vi "MeasureGrowthNotLog.vi"(10 "DaysBack":i32=7, 11 "Data":cluster{"Cases":i32[], "Days":timestamp[]}={"Cases"=[0, 0, 0, 0, 2, 2, 2, 2, 2, 3, 3, 3, 6, 6, 6, 6, 6, 6, 6, 6, 7, 7, 8, 8, 8, 8, 8, 8, 8, 8, 10, 10, 10, 10, 10, 10, 11, 11, 12, 12, 21, 25, 35, 51, 59, 102, 116, 167, 179, 247, 250, 305, 372, 480, 588, 741, 892, 1065, 1289, 1524, 1826, 2253, 2641, 3176, 4035, 4863, 5671, 6352, 7412, 8570, 9939, 11170, 12563, 13886], "Days"=[timestamp(3662524800 s since 1904-01-01), timestamp(3662611200 s since 1904-01-01), timestamp(3662697600 s since 1904-01-01), timestamp(3662784000 s since 1904-01-01), timestamp(3662870400 s since 1904-01-01), timestamp(3662956800 s since 1904-01-01), timestamp(3663043200 s since 1904-01-01), timestamp(3663129600 s since 1904-01-01), timestamp(3663216000 s since 1904-01-01), timestamp(3663302400 s since 1904-01-01), timestamp(3663388800 s since 1904-01-01), timestamp(3663475200 s since 1904-01-01), timestamp(3663561600 s since 1904-01-01), timestamp(3663648000 s since 1904-01-01), timestamp(3663734400 s since 1904-01-01), timestamp(3663820800 s since 1904-01-01), timestamp(3663907200 s since 1904-01-01), timestamp(3663993600 s since 1904-01-01), timestamp(3664080000 s since 1904-01-01), timestamp(3664166400 s since 1904-01-01), timestamp(3664252800 s since 1904-01-01), timestamp(3664339200 s since 1904-01-01), timestamp(3664425600 s since 1904-01-01), timestamp(3664512000 s since 1904-01-01), timestamp(3664598400 s since 1904-01-01), timestamp(3664684800 s since 1904-01-01), timestamp(3664771200 s since 1904-01-01), timestamp(3664857600 s since 1904-01-01), timestamp(3664944000 s since 1904-01-01), timestamp(3665030400 s since 1904-01-01), timestamp(3665116800 s since 1904-01-01), timestamp(3665203200 s since 1904-01-01), timestamp(3665289600 s since 1904-01-01), timestamp(3665376000 s since 1904-01-01), timestamp(3665462400 s since 1904-01-01), timestamp(3665548800 s since 1904-01-01), timestamp(3665635200 s since 1904-01-01), timestamp(3665721600 s since 1904-01-01), timestamp(3665808000 s since 1904-01-01), timestamp(3665894400 s since 1904-01-01), timestamp(3665980800 s since 1904-01-01), timestamp(3666067200 s since 1904-01-01), timestamp(3666153600 s since 1904-01-01), timestamp(3666240000 s since 1904-01-01), timestamp(3666326400 s since 1904-01-01), timestamp(3666412800 s since 1904-01-01), timestamp(3666499200 s since 1904-01-01), timestamp(3666585600 s since 1904-01-01), timestamp(3666672000 s since 1904-01-01), timestamp(3666758400 s since 1904-01-01), timestamp(3666844800 s since 1904-01-01), timestamp(3666931200 s since 1904-01-01), timestamp(3667017600 s since 1904-01-01), timestamp(3667104000 s since 1904-01-01), timestamp(3667190400 s since 1904-01-01), timestamp(3667276800 s since 1904-01-01), timestamp(3667363200 s since 1904-01-01), timestamp(3667449600 s since 1904-01-01), timestamp(3667536000 s since 1904-01-01), timestamp(3667622400 s since 1904-01-01), timestamp(3667708800 s since 1904-01-01), timestamp(3667795200 s since 1904-01-01), timestamp(3667881600 s since 1904-01-01), timestamp(3667968000 s since 1904-01-01), timestamp(3668054400 s since 1904-01-01), timestamp(3668140800 s since 1904-01-01), timestamp(3668227200 s since 1904-01-01), timestamp(3668313600 s since 1904-01-01), timestamp(3668400000 s since 1904-01-01), timestamp(3668486400 s since 1904-01-01), timestamp(3668572800 s since 1904-01-01), timestamp(3668659200 s since 1904-01-01), timestamp(3668745600 s since 1904-01-01), timestamp(3668832000 s since 1904-01-01)]}) -> (0 "Plot":T2(graph)=[{"Days"=[timestamp(3662524800 s since 1904-01-01), timestamp(3662611200 s since 1904-01-01), timestamp(3662697600 s since 1904-01-01), timestamp(3662784000 s since 1904-01-01), timestamp(3662870400 s since 1904-01-01), timestamp(3662956800 s since 1904-01-01), timestamp(3663043200 s since 1904-01-01), timestamp(3663129600 s since 1904-01-01), timestamp(3663216000 s since 1904-01-01), timestamp(3663302400 s since 1904-01-01), timestamp(3663388800 s since 1904-01-01), timestamp(3663475200 s since 1904-01-01), timestamp(3663561600 s since 1904-01-01), timestamp(3663648000 s since 1904-01-01), timestamp(3663734400 s since 1904-01-01), timestamp(3663820800 s since 1904-01-01), timestamp(3663907200 s since 1904-01-01), timestamp(3663993600 s since 1904-01-01), timestamp(3664080000 s since 1904-01-01), timestamp(3664166400 s since 1904-01-01), timestamp(3664252800 s since 1904-01-01), timestamp(3664339200 s since 1904-01-01), timestamp(3664425600 s since 1904-01-01), timestamp(3664512000 s since 1904-01-01), timestamp(3664598400 s since 1904-01-01), timestamp(3664684800 s since 1904-01-01), timestamp(3664771200 s since 1904-01-01), timestamp(3664857600 s since 1904-01-01), timestamp(3664944000 s since 1904-01-01), timestamp(3665030400 s since 1904-01-01), timestamp(3665116800 s since 1904-01-01), timestamp(3665203200 s since 1904-01-01), timestamp(3665289600 s since 1904-01-01), timestamp(3665376000 s since 1904-01-01), timestamp(3665462400 s since 1904-01-01), timestamp(3665548800 s since 1904-01-01), timestamp(3665635200 s since 1904-01-01), timestamp(3665721600 s since 1904-01-01), timestamp(3665808000 s since 1904-01-01), timestamp(3665894400 s since 1904-01-01), timestamp(3665980800 s since 1904-01-01), timestamp(3666067200 s since 1904-01-01), timestamp(3666153600 s since 1904-01-01), timestamp(3666240000 s since 1904-01-01), timestamp(3666326400 s since 1904-01-01), timestamp(3666412800 s since 1904-01-01), timestamp(3666499200 s since 1904-01-01), timestamp(3666585600 s since 1904-01-01), timestamp(3666672000 s since 1904-01-01), timestamp(3666758400 s since 1904-01-01), timestamp(3666844800 s since 1904-01-01), timestamp(3666931200 s since 1904-01-01), timestamp(3667017600 s since 1904-01-01), timestamp(3667104000 s since 1904-01-01), timestamp(3667190400 s since 1904-01-01), timestamp(3667276800 s since 1904-01-01), timestamp(3667363200 s since 1904-01-01), timestamp(3667449600 s since 1904-01-01), timestamp(3667536000 s since 1904-01-01), timestamp(3667622400 s since 1904-01-01), timestamp(3667708800 s since 1904-01-01), timestamp(3667795200 s since 1904-01-01), timestamp(3667881600 s since 1904-01-01), timestamp(3667968000 s since 1904-01-01), timestamp(3668054400 s since 1904-01-01), timestamp(3668140800 s since 1904-01-01), timestamp(3668227200 s since 1904-01-01), timestamp(3668313600 s since 1904-01-01), timestamp(3668400000 s since 1904-01-01), timestamp(3668486400 s since 1904-01-01), timestamp(3668572800 s since 1904-01-01), timestamp(3668659200 s since 1904-01-01), timestamp(3668745600 s since 1904-01-01), timestamp(3668832000 s since 1904-01-01)], "ConfirmedCases"=[0.0, 0.0, 0.0, 0.0, 0.0, 0.0, 0.0, 0.0, 0.0, 0.0, 0.0, 0.0, 0.0, 0.0, 0.0, 0.0, 0.0, 0.0, 0.0, 0.0, 0.0, 0.0, 0.0, 0.0, 0.0, 0.0, 0.0, 0.0, 0.0, 0.0, 0.0, 0.0, 0.0, 0.0, 0.0, 0.0, 0.0, 0.0, 0.0, 0.0, 0.0, 0.0, 1.0, 1.0, 1.0, 1.0, 1.0, 2.0, 3.0, 4.0, 4.0, 4.0, 4.0, 6.0, 11.0, 14.0, 17.0, 19.0, 24.0, 29.0, 33.0, 40.0, 52.0, 67.0, 83.0, 100.0, 121.0, 132.0, 149.0, 182.0, 212.0, 243.0, 282.0, 321.0]}, {"Days"=[timestamp(3668313600 s since 1904-01-01), timestamp(3668400000 s since 1904-01-01), timestamp(3668486400 s since 1904-01-01), timestamp(3668572800 s since 1904-01-01), timestamp(3668659200 s since 1904-01-01), timestamp(3668745600 s since 1904-01-01), timestamp(3668832000 s since 1904-01-01)], "ConfirmedCases"=[132.01823524302534, 153.55263572024907, 178.59966006386384, 207.73227646213113, 241.6169138771523, 281.0287070731711, 326.8692283660796]}, {"Days"=[timestamp(3668313600 s since 1904-01-01), timestamp(3668400000 s since 1904-01-01), timestamp(3668486400 s since 1904-01-01), timestamp(3668572800 s since 1904-01-01), timestamp(3668659200 s since 1904-01-01), timestamp(3668745600 s since 1904-01-01), timestamp(3668832000 s since 1904-01-01)], "ConfirmedCases"=[140.59609548662908, 162.8828644131387, 188.9766356577397, 219.6124606618654, 255.65531024069676, 298.10468948116306, 348.1074955925532]}, {"Days"=[timestamp(3668313600 s since 1904-01-01), timestamp(3668400000 s since 1904-01-01), timestamp(3668486400 s since 1904-01-01), timestamp(3668572800 s since 1904-01-01), timestamp(3668659200 s since 1904-01-01), timestamp(3668745600 s since 1904-01-01), timestamp(3668832000 s since 1904-01-01)], "ConfirmedCases"=[123.96371589380509, 144.75685960943596, 168.7924989452066, 196.49476425010758, 228.34938580605382, 264.9308682016178, 306.9267217896756]}, {"Days"=[timestamp(3668313600 s since 1904-01-01), timestamp(3668400000 s since 1904-01-01), timestamp(3668486400 s since 1904-01-01), timestamp(3668572800 s since 1904-01-01), timestamp(3668659200 s since 1904-01-01), timestamp(3668745600 s since 1904-01-01), timestamp(3668832000 s since 1904-01-01)], "ConfirmedCases"=[140.59609548662908, 160.133980854025, 182.38694136848164, 207.73227646213113, 236.5997168457177, 269.47871060219524, 306.9267217896756]}, {"Days"=[timestamp(3668313600 s since 1904-01-01), timestamp(3668400000 s since 1904-01-01), timestamp(3668486400 s since 1904-01-01), timestamp(3668572800 s since 1904-01-01), timestamp(3668659200 s since 1904-01-01), timestamp(3668745600 s since 1904-01-01), timestamp(3668832000 s since 1904-01-01)], "ConfirmedCases"=[123.96371589380509, 147.24177723483396, 174.89102199747728, 207.73227646213113, 246.7405026929383, 293.0737423477007, 348.1074955925532]}], 1 "Interval":dbl, 2 "PlusMinus":dbl=2.4408305776857144, 3 "Growth":dbl=16.31168636482856, 4 "GrowthLower":dbl=13.896463696073248, 5 "Measure":T1={"Trend"=0.0, "TrendBest"=0.0, "TrendWorst"=0.0, "BestDays"=0.0, "WorstDays"=0.0, "Days"=0.0, "Growth"=16.31168636482856, "PlusMinus"=2.4408305776857144, "Cases"=0}, 6 "GrowthUpper":dbl=18.778124851444677)   [LabVIEW 2017]
uses:
  <vilib>/Analysis/6fits.llb/Prediction Interval (Linear).vi
  <vilib>/Analysis/1siggen.llb/Ramp Pattern by Samples.vi
  <vilib>/Analysis/NI_AALPro.lvlib
  <vilib>/Analysis/NI_AALBase.lvlib
panel:
  out "Days":dbl
  out "WorstDays":dbl
  out "BestDays":dbl
  out "TrendWorst":dbl
  out "TrendBest":dbl
  out "Trend":dbl
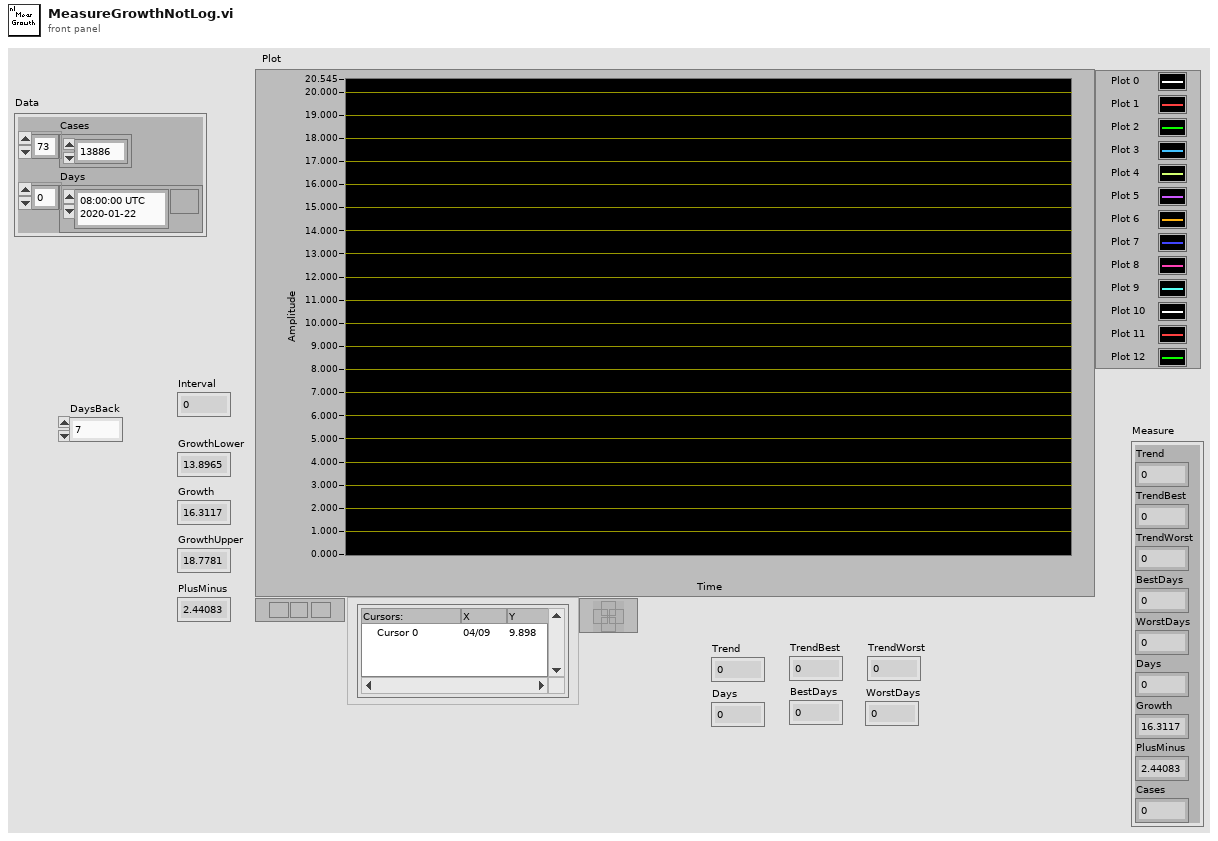
[diagram p1: front panel]
types:
  T1 = cluster{"Trend":dbl, "TrendBest":dbl, "TrendWorst":dbl, "BestDays":dbl, "WorstDays":dbl, "Days":dbl, "Growth":dbl, "PlusMinus":dbl, "Cases":i32}
  T2 = cluster{"Days":timestamp[], "ConfirmedCases":dbl[]}[]
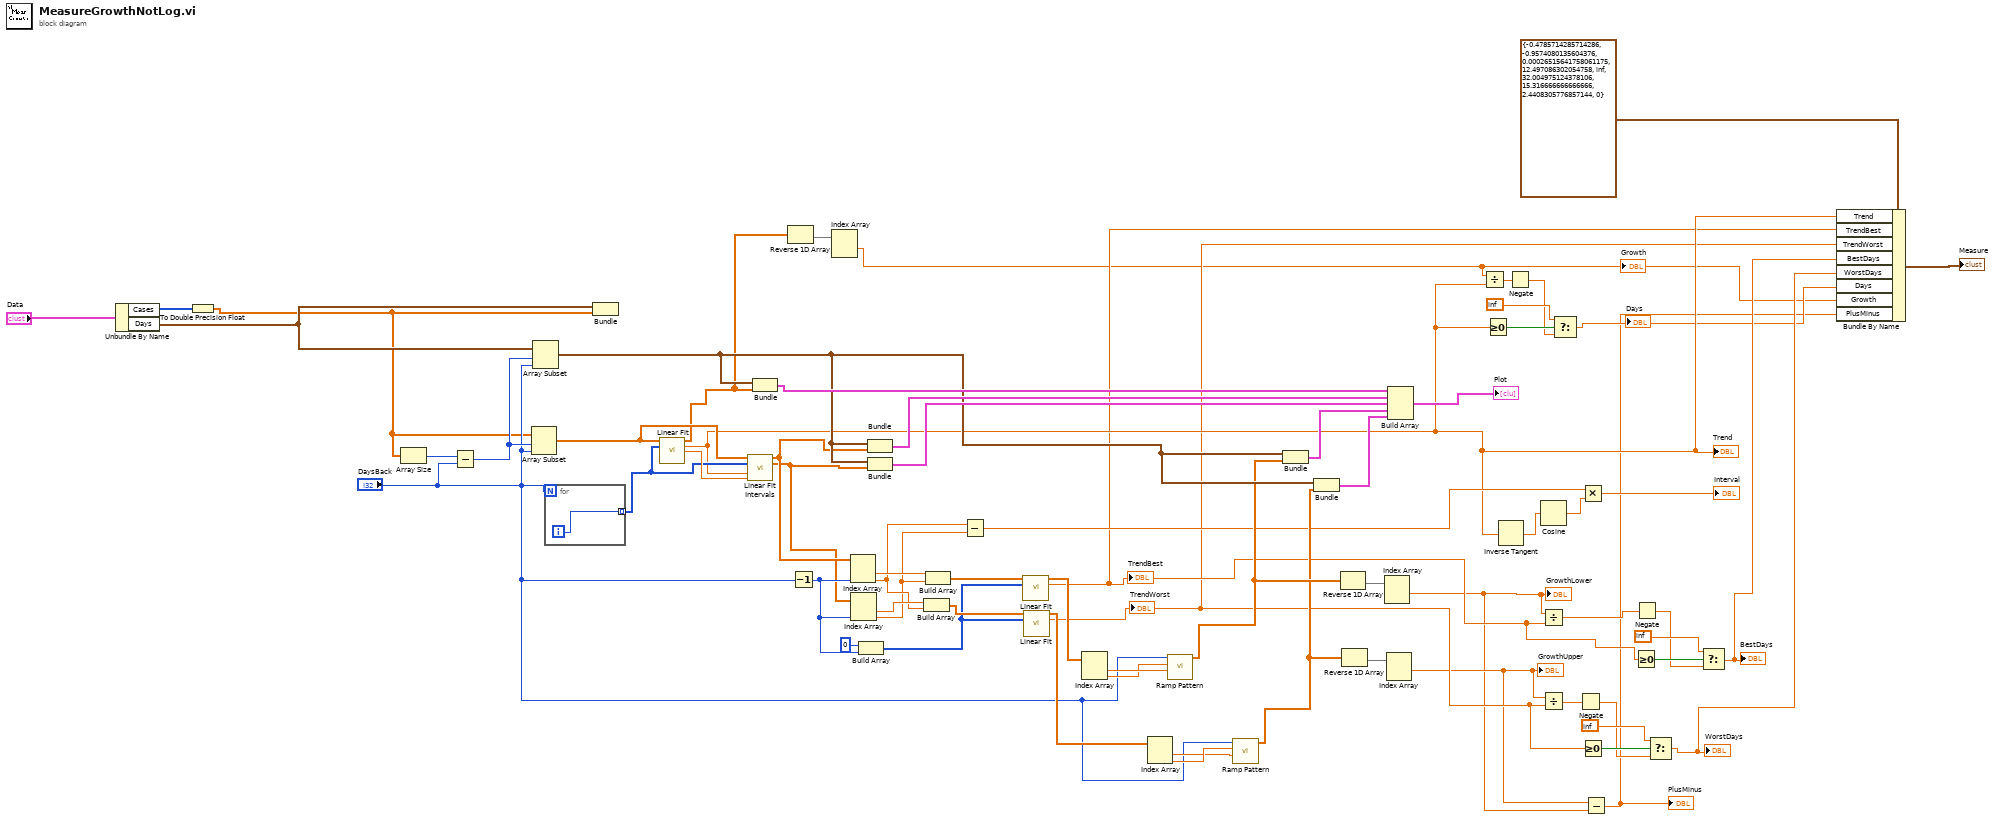
[diagram p0: block diagram]
diagram:
  n1 = Unbundle By Name("Data") -> ("Cases"=w32:i32[], "Days"=w40:timestamp[])
  n2 = To Double Precision Float(number=w32) -> (double precision float=w31:dbl[])
  n3 = Array Size(array=w31) -> (size(s)=w68:i32)
  n4 = Subtract(x=w68, y="DaysBack") -> (x-y=w67:i32)
  n5 = Array Subset(array=w31, index=w67, length="DaysBack") -> (w42:dbl[])
  n6 = Array Subset(array=w40, index=w67, length="DaysBack") -> (w39:timestamp[])
  n7 = for {
    N: "DaysBack" -> [_]
    tunnel: [w69] -> w41 mode=indexing
    i -> [w69]
  }
  n8 = Bundle("Days"=w40, w31) -> ()  [unwired: 1 in, 1 out]
  n9 = call <vilib>:"Linear Fit.vi"("Y"=w42, "X"=w41) -> ("Best Linear Fit"=w37:dbl[], "slope"=w11:dbl, "intercept"=w65:dbl)  [unwired: 9 in, 2 out]
  "Trend" <- w11
  n10 = call-poly <vilib>:"Linear Fit Intervals.vi"("Y"=w42, "X"=w41, "slope"=w11, "intercept"=w65) -> ("Upper Bound"=w36:dbl[], "Lower Bound"=w35:dbl[])  [unwired: 9 in, 1 out]
  n11 = Bundle(w39, "Best Linear Fit"=w37) -> (w66:cluster{timestamp[], "Best Linear Fit":dbl[]})  [unwired: 1 in]
  n12 = Reverse 1D Array(array=w37) -> (reversed array=w61:dbl[])
  n13 = Decrement(x="DaysBack") -> (x-1=w57:i32)
  n14 = Index Array(array=w61) -> (element #1=w5:dbl)  [unwired: 2 in, 1 out]
  "Growth" <- w5
  n15 = Index Array(array=w36, index #2=w57) -> (element #1=w59:dbl, element #2=w30:dbl)  [unwired: 1 in]
  n16 = Index Array(array=w35, index #2=w57) -> (element #1=w54:dbl, element #2=w29:dbl)  [unwired: 1 in]
  n17 = Build Array(0 ("element"), w57) -> (w55:i32[])
  n18 = Bundle(w39, "Upper Bound"=w36) -> (w64:cluster{timestamp[], "Upper Bound":dbl[]})  [unwired: 1 in]
  n19 = Bundle(w39, "Lower Bound"=w35) -> (w63:cluster{timestamp[], "Lower Bound":dbl[]})  [unwired: 1 in]
  n20 = Build Array(w54, w30) -> (w56:dbl[])
  n21 = Build Array(w59, w29) -> (w58:dbl[])
  n22 = Subtract(x=w30, y=w29) -> (x-y=w27:dbl)
  n23 = call <vilib>:"Linear Fit.vi"("Y"=w58, "X"=w55) -> ("Best Linear Fit"=w53:dbl[], "slope"=w10:dbl)  [unwired: 9 in, 3 out]
  "TrendBest" <- w10
  n24 = call <vilib>:"Linear Fit.vi"("Y"=w56, "X"=w55) -> ("Best Linear Fit"=w48:dbl[], "slope"=w9:dbl)  [unwired: 9 in, 3 out]
  "TrendWorst" <- w9
  n25 = Index Array(array=w53) -> (element #1=w52:dbl, element #2=w51:dbl)  [unwired: 2 in]
  n26 = Index Array(array=w48) -> (element #1=w49:dbl, element #2=w50:dbl)  [unwired: 2 in]
  n27 = call-poly <vilib>:"Ramp Pattern.vi"("start"=w52, "end"=w51, "samples"="DaysBack") -> ("Ramp Pattern"=w34:dbl[])  [unwired: 7 in, 1 out]
  n28 = call-poly <vilib>:"Ramp Pattern.vi"("start"=w49, "end"=w50, "samples"="DaysBack") -> ("Ramp Pattern"=w33:dbl[])  [unwired: 7 in, 1 out]
  n29 = Bundle(w39, "Ramp Pattern"=w34) -> (w46:cluster{timestamp[], "Ramp Pattern":dbl[]})  [unwired: 1 in]
  n30 = Bundle(w39, "Ramp Pattern"=w33) -> (w45:cluster{timestamp[], "Ramp Pattern":dbl[]})  [unwired: 1 in]
  n31 = Reverse 1D Array(array=w34) -> (reversed array=w44:dbl[])
  n32 = Reverse 1D Array(array=w33) -> (reversed array=w43:dbl[])
  n33 = Index Array(array=w44) -> (element #1=w3:dbl)  [unwired: 2 in, 1 out]
  "GrowthLower" <- w3
  n34 = Index Array(array=w43) -> (element #1=w4:dbl)  [unwired: 2 in, 1 out]
  "GrowthUpper" <- w4
  n35 = Build Array(w66, w64, w63, w46, w45) -> (→"Plot":cluster{timestamp[], "Ramp Pattern":dbl[]}[])
  n36 = Divide(x=w5, y=w11) -> (x/y=w18:dbl)
  n37 = Greater Or Equal To 0?(x=w11) -> (x >= 0?=w24:bool)
  n38 = Inverse Tangent(1:w11) -> (0:w28:dbl)
  n39 = Negate(x=w18) -> (-x=w17:dbl)
  n40 = Cosine(x=w28) -> (cos(x)=w26:dbl)
  n41 = Divide(x=w3, y=w10) -> (x/y=w16:dbl)
  n42 = Divide(x=w4, y=w9) -> (x/y=w14:dbl)
  n43 = Select(t=inf, s=w24, f=w17) -> (s? t:f=w6:dbl)
  "Days" <- w6
  n44 = Negate(x=w14) -> (-x=w13:dbl)
  n45 = Multiply(x=w27, y=w26) -> (x*y=→"Interval":dbl)
  n46 = Greater Or Equal To 0?(x=w9) -> (x >= 0?=w22:bool)
  n47 = Subtract(x=w4, y=w3) -> (x-y=w2:dbl)
  "PlusMinus" <- w2
  n48 = Greater Or Equal To 0?(x=w10) -> (x >= 0?=w19:bool)
  n49 = Negate(x=w16) -> (-x=w15:dbl)
  n50 = Select(t=inf, s=w22, f=w13) -> (s? t:f=w7:dbl)
  "WorstDays" <- w7
  n51 = Select(t=inf, s=w19, f=w15) -> (s? t:f=w8:dbl)
  "BestDays" <- w8
  n52 = Bundle By Name(cluster=T1 {"Trend"=-0.4785714285714286, "TrendBest"=-0.9574080135604376, "TrendWorst"=0.00026515641758061175, "BestDays"=12.497086302054758, "WorstDays"=inf, "Days"=32.004975124378106, "Growth"=15.316666666666666, "PlusMinus"=2.4408305776857144, "Cases"=0} ("Measure"), "Trend"=w11, "TrendBest"=w10, "TrendWorst"=w9, "BestDays"=w8, "WorstDays"=w7, "Days"=w6, "Growth"=w5, "PlusMinus"=w2) -> (→"Measure":T1)
